vi "Butterfly_PullDown RCV_TTR.vi"(0 "Semiconductor Module Context":T2, 1 "RFPins":string[](array[string]), 3 "R Thresholds":dbl[](array[numeric]), 4 "Capacitance":bool=TRUE, 5 "error in (no error)":errorcluster, 6 "VNAs Measurement Parameters":T1, 7 "Start_v":dbl=10.0 format="%#_13g", 8 "C_TH_Delta":dbl=2.0, 9 "Stop_v":dbl=41.0 format="%#_13g", 10 "PD_Pin":string="SMU_PD", 11 "Step_v":dbl=1.0) -> (14 "Semiconductor Module Context Out":T2, 19 "error out":errorcluster)   [LabVIEW 2013]
uses:
  <vilib>/NI_TestStand_SemiconductorModule/NI_TestStand_Semiconductor_Module.lvlibp/PinMap/General/SemiconductorModuleContext.ctl
  VNA/VNAs Measurement Parameters.ctl
  <instrlib>/niDCPower/nidcpower.llb/niDCPower Wait For Event - Event.ctl
  <vilib>/NI_TestStand_SemiconductorModule/NI_TestStand_Semiconductor_Module.lvlibp/PinMap/DC Power/PinToNIDCPowerSession.vi
  <vilib>/NI_TestStand_SemiconductorModule/NI_TestStand_Semiconductor_Module.lvlibp/PinMap/DC Power/PinsToNIDCPowerSessions.vi
  <vilib>/NI_TestStand_SemiconductorModule/NI_TestStand_Semiconductor_Module.lvlibp/PinMap/General/Publish/PublishDataDoubleFunctionalTest.vi
  <vilib>/NI_TestStand_SemiconductorModule/NI_TestStand_Semiconductor_Module.lvlibp/PinMap/General/Publish/PublishDataDouble2D.vi
  <vilib>/NI_TestStand_SemiconductorModule/NI_TestStand_Semiconductor_Module.lvlibp
  VNA/Pin Map API/VNA Custom Instrument.lvlib
panel:
  in  "current level":dbl=0.01 format="%_6p"
  out "VPIs 2":dbl[](array[numeric])
  out "VRLs 2":dbl[](array[numeric])
  out "S0 steps":dbl[](array[numeric]) format="%#_3g"
  out "S1 steps":dbl[](array[numeric]) format="%#_3g"
  out "S2 steps":dbl[](array[numeric]) format="%#_3g"
  out "S3 steps":dbl[](array[numeric]) format="%#_3g"
  out "appended array":dbl[][](array[numeric]) format="%#_3g"
  out "VPIs":dbl[][](array[numeric]) format="%#_3g"
  out "VRLs":dbl[][](array[numeric]) format="%#_3g"
  out "C_Free":dbl[](array[numeric])
  out "Full R Array":dbl[][][](array[numeric])
  out "step":i32
  out "sites and pins loop iter":i32
  out "BF values":dbl[](array[numeric])
  out "BF Names":string[](array[string])
  out "R Array":dbl[](array[numeric])
  out "BFSamples":i32
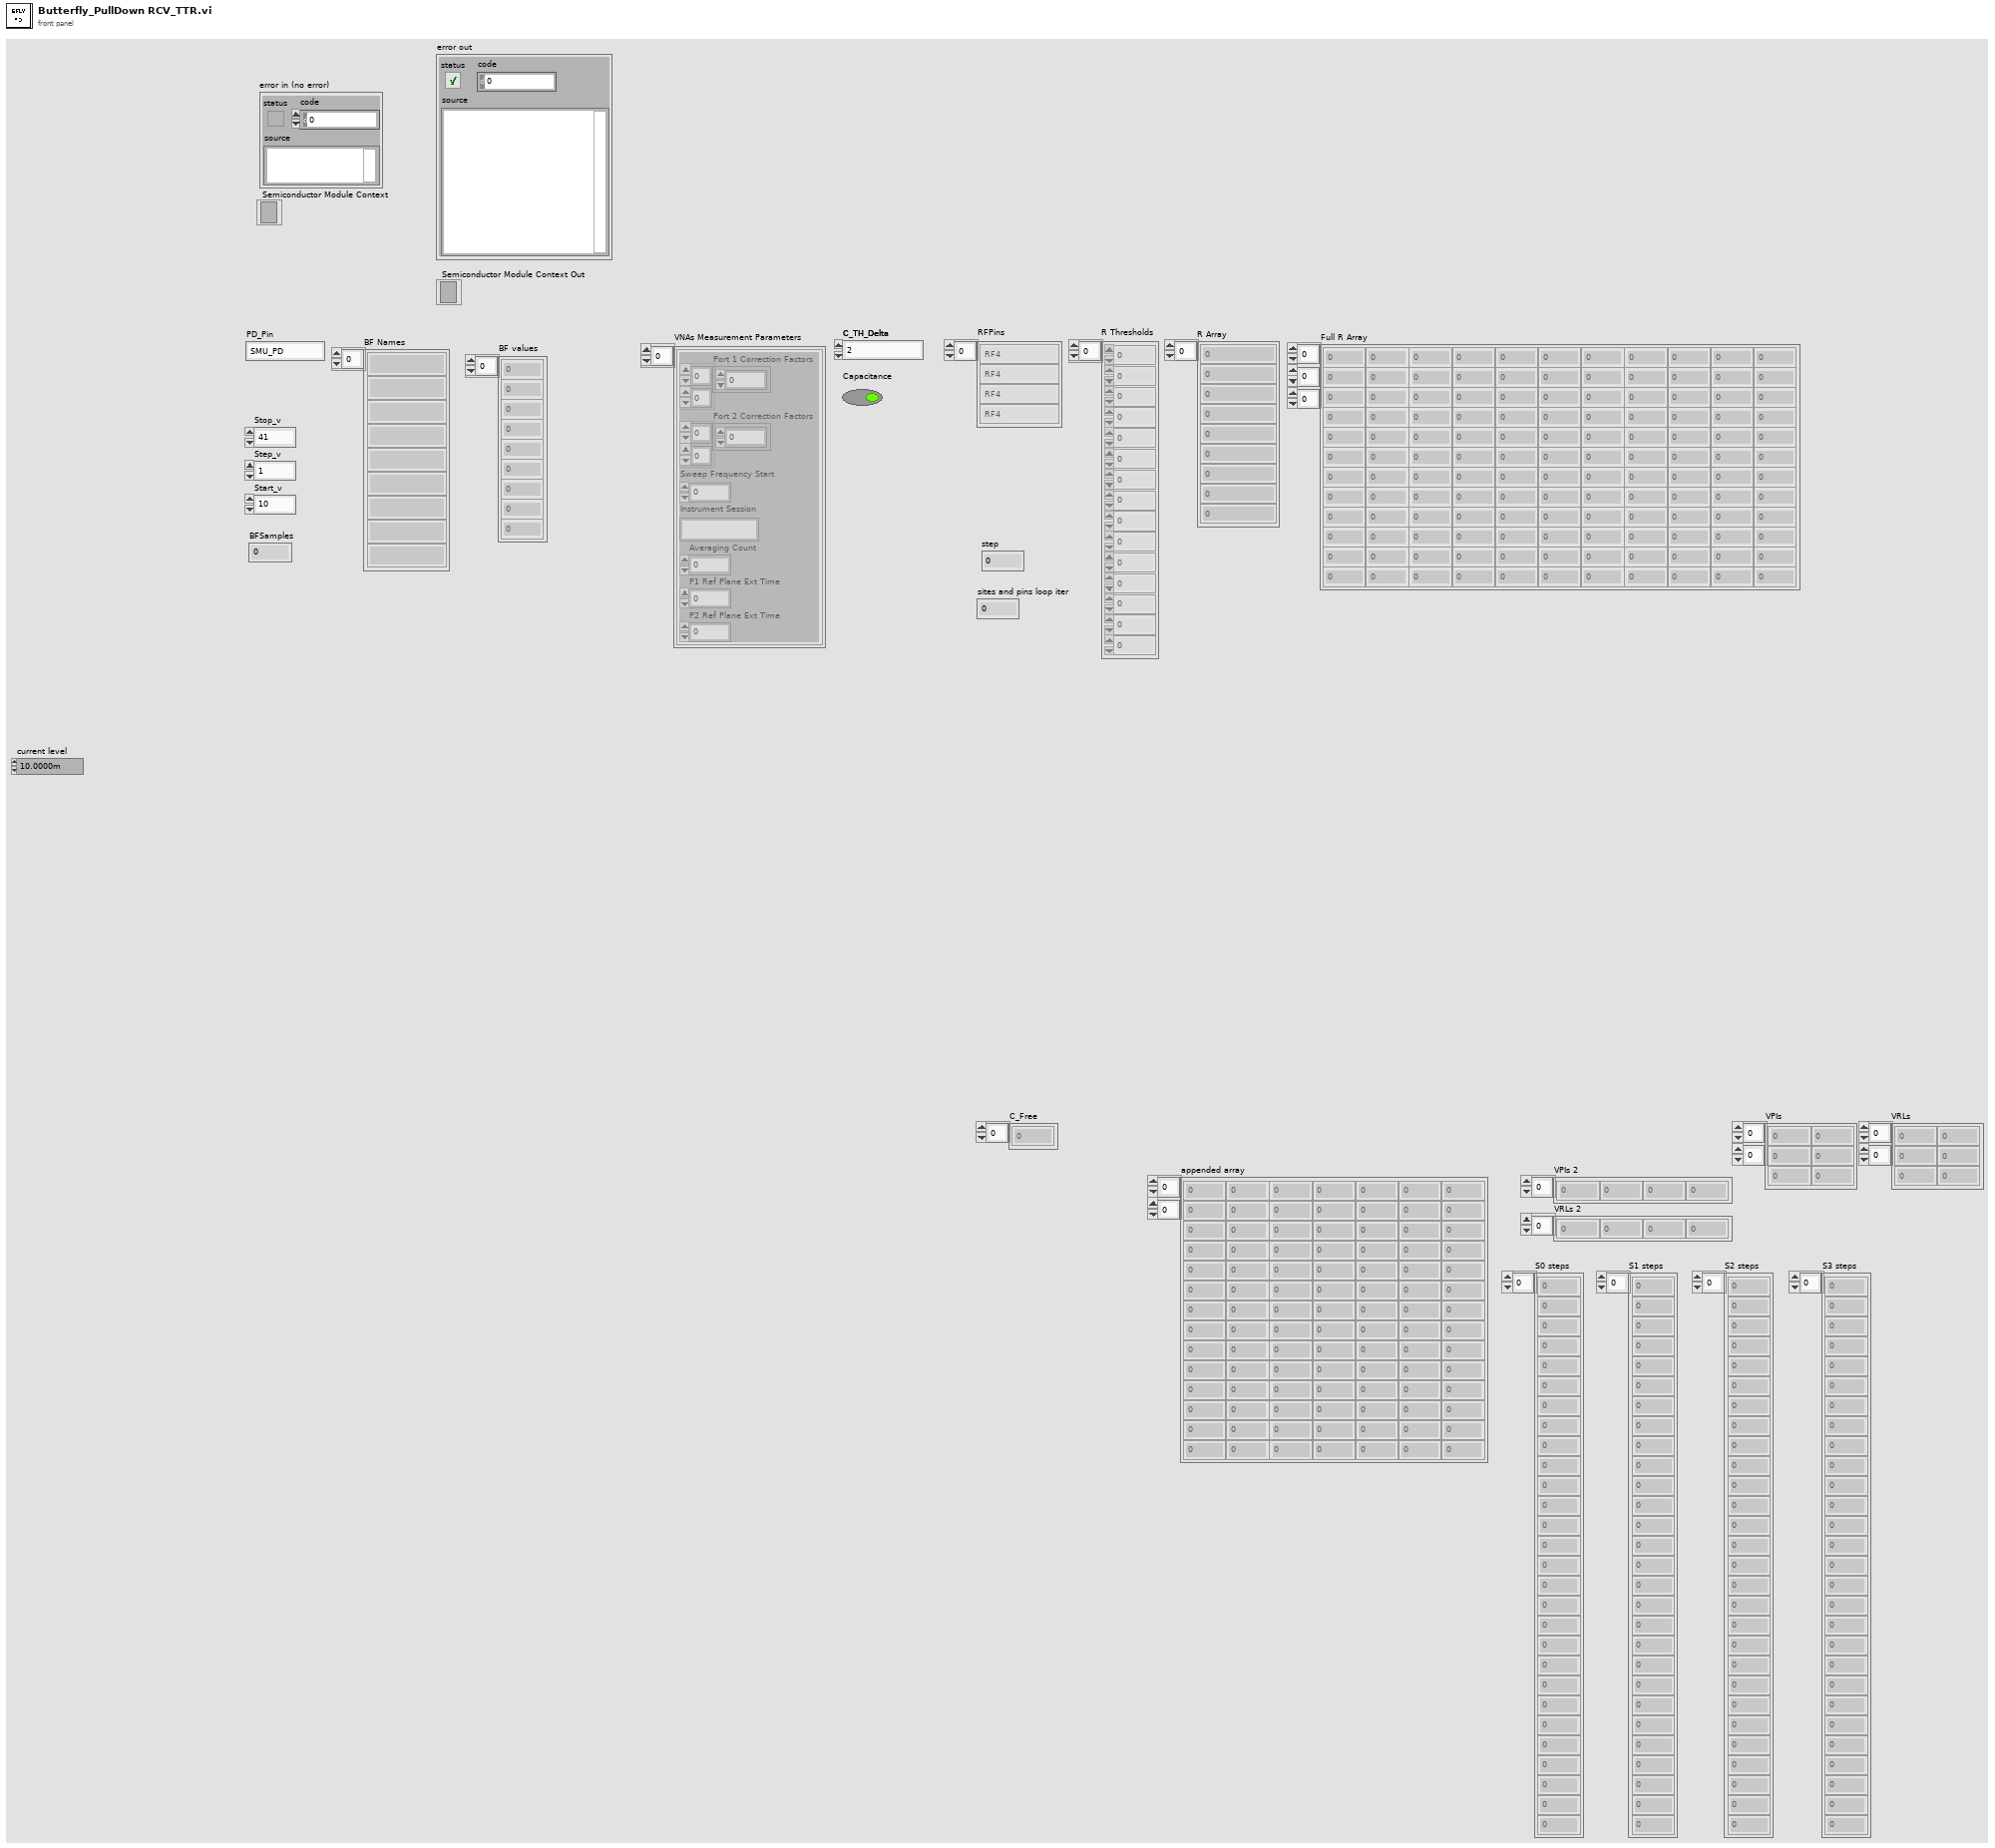
[diagram p1: front panel]
types:
  T1 = typedef "VNAs Measurement Parameters.ctl" = cluster{"Port 1 Correction Factors":cdb[][], "Port 2 Correction Factors":cdb[][], "Sweep Frequency Start":dbl, "Instrument Session":string, "Averaging Count":i32, "P1 Ref Plane Ext Time":dbl, "P2 Ref Plane Ext Time":dbl}[]
  T2 = typedef "NI_TestStand_Semiconductor_Module.lvlibp/SemiconductorModuleContext.ctl" = refnum<k7>
  T3 = typedef "niDCPower Wait For Event - Event.ctl" = i32
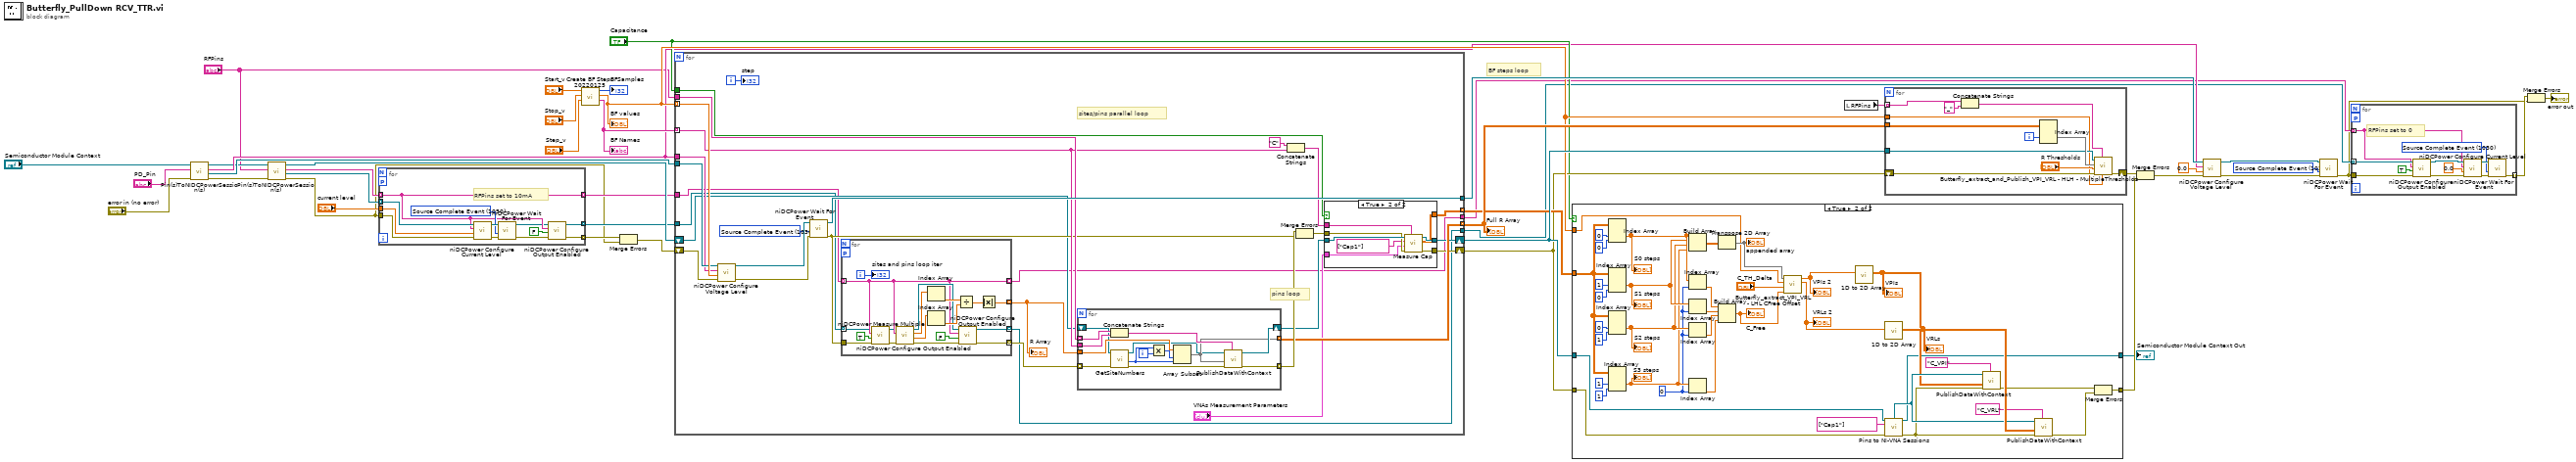
[diagram p0: block diagram]
diagram:
  w35 = T3 1030 items=["Source Complete Event"=1030, "Measure Complete Event"=1031, "Sequence Iteration Complete Event"=1032, "Sequence Engine Done Event"=1033, "Pulse Complete Event"=1051, "Ready For Pulse Trigger Event"=1052] ("event")
  # "BF steps loop"
  n1 = call-poly <vilib>:"Pin(s)ToNIDCPowerSession(s).vi"("error in (no error)"="error in (no error)", "Pin"="PD_Pin", "Semiconductor Module Context"="Semiconductor Module Context") -> ("error out"=w17:errorcluster, "Instrument Session"=w19:refnum<k15>, "Channel List"=w18:string, "Semiconductor Module Context Out"=w16:T2)  [unwired: 4 in, 1 out]
  n2 = call-poly <vilib>:"Pin(s)ToNIDCPowerSession(s).vi"("error in (no error)"=w17, "Pins"="RFPins", "Semiconductor Module Context"=w16) -> ("error out"=w1:errorcluster, "Instrument Sessions"=w13:refnum<k15>[], "Channel Lists"=w12:string[], "Semiconductor Module Context Out"=w15:T2)  [unwired: 4 in, 1 out]
  n3 = for {
    tunnel: w13 -> [w53] mode=indexing
    tunnel: w12 -> [w46] mode=indexing
    tunnel: "current level" -> [w50]
    tunnel: [w47] -> w9 mode=indexing
    tunnel: [w46] -> w10 mode=indexing
    workers-P: _ -> [_]
    tunnel: w1 -> [w52]
    tunnel: [w49] -> w2 mode=indexing
    w51 = T3 1030 items=["Source Complete Event"=1030, "Measure Complete Event"=1031, "Sequence Iteration Complete Event"=1032, "Sequence Engine Done Event"=1033, "Pulse Complete Event"=1051, "Ready For Pulse Trigger Event"=1052] ("event")
    # "RFPins set to 10mA"
    n4 = call <instrlib>:"niDCPower Configure Current Level.vi"("error in (no error)"=w52, "current level"=w50, "channel name"=w46, "instrument handle"=w53) -> ("error out"=w55:errorcluster, "instrument handle out"=w54:refnum<k15>)  [unwired: 6 in]
    n5 = call <instrlib>:"niDCPower Wait For Event.vi"("error in (no error)"=w55, "event"=w51, "instrument handle"=w54) -> ("error out"=w44:errorcluster, "instrument handle out"=w45:refnum<k15>)  [unwired: 7 in]
    n6 = call <instrlib>:"niDCPower Configure Output Enabled.vi"("error in (no error)"=w44, "output enabled"=FALSE, "channel name"=w46, "instrument handle"=w45) -> ("error out"=w49:errorcluster, "instrument handle out"=w47:refnum<k15>)  [unwired: 6 in]
  }
  n7 = call "Create BF Steps 20220125.vi"("Step_v"="Step_v", "Stop_v"="Stop_v", "Start_v"="Start_v") -> ("BF Names"=w34:string[], "BF values"=w29:dbl[], "BFSamples"=→"BFSamples":i32)  [unwired: 6 in]
  "BF Names" <- w34
  "BF values" <- w29
  n8 = Merge Errors(w2, w1) -> (w3:errorcluster)
  n9 = for {
    shift-right: [w69] -> w28
    shift-left: w3 -> [w82]
    tunnel: w29 -> [w81] mode=indexing
    tunnel: w19 -> [w80]
    tunnel: [w79] -> w38
    shift-right: [w64] -> w31
    shift-left: w15 -> [w60]
    tunnel: "RFPins" -> [w76]
    tunnel: w34 -> [w67] mode=indexing
    tunnel: [w74] -> w32 mode=indexing
    tunnel: "Capacitance" -> [w65]
    tunnel: [w63] -> w30 mode=indexing
    tunnel: w18 -> [w62]
    tunnel: w10 -> [w59]
    tunnel: w9 -> [w58]
    tunnel: [w57] -> w8
    tunnel: [w56] -> w7
    i -> [w78]
    w84 = T3 1030 items=["Source Complete Event"=1030, "Measure Complete Event"=1031, "Sequence Iteration Complete Event"=1032, "Sequence Engine Done Event"=1033, "Pulse Complete Event"=1051, "Ready For Pulse Trigger Event"=1052] ("event")
    # "pins loop"
    # "sites/pins parallel loop"
    n10 = call <instrlib>:"niDCPower Configure Voltage Level.vi"("error in (no error)"=w82, "voltage level"=w81, "channel name"=w62, "instrument handle"=w80) -> ("error out"=w83:errorcluster, "instrument handle out"=w85:refnum<k15>)  [unwired: 6 in]
    n11 = call <instrlib>:"niDCPower Wait For Event.vi"("error in (no error)"=w83, "event"=w84, "instrument handle"=w85) -> ("error out"=w61:errorcluster, "instrument handle out"=w79:refnum<k15>)  [unwired: 7 in]
    n12 = for {
      tunnel: w61 -> [w120]
      tunnel: [w122] -> w75 mode=indexing
      tunnel: [w117] -> w73 mode=indexing
      workers-P: _ -> [_]
      tunnel: w59 -> [w114] mode=indexing
      tunnel: w58 -> [w113] mode=indexing
      tunnel: [w115] -> w57 mode=indexing
      tunnel: [w114] -> w56 mode=indexing
      i -> [w121]
      n13 = call <instrlib>:"niDCPower Configure Output Enabled.vi"("error in (no error)"=w120, "output enabled"=TRUE, "channel name"=w114, "instrument handle"=w113) -> ("error out"=w119:errorcluster, "instrument handle out"=w110:refnum<k15>)  [unwired: 6 in]
      n14 = call <instrlib>:"niDCPower Measure Multiple.vi"("error in (no error)"=w119, "channel name"=w114, "instrument handle"=w110) -> ("error out"=w118:errorcluster, "current measurements"=w123:dbl[], "voltage measurements"=w124:dbl[], "instrument handle out"=w116:refnum<k15>)  [unwired: 5 in]
      n15 = Index Array(array=w124) -> (element=w126:dbl)  [unwired: 1 in]
      n16 = Index Array(array=w123) -> (element=w125:dbl)  [unwired: 1 in]
      n17 = Divide(x=w126, y=w125) -> (x/y=w127:dbl)
      n18 = call <instrlib>:"niDCPower Configure Output Enabled.vi"("error in (no error)"=w118, "output enabled"=FALSE, "channel name"=w114, "instrument handle"=w116) -> ("error out"=w117:errorcluster, "instrument handle out"=w115:refnum<k15>)  [unwired: 6 in]
      n19 = Absolute Value(x=w127) -> (abs(x)=w122:dbl)
      "sites and pins loop iter" <- w121
    }
    "R Array" <- w75
    n20 = for {
      tunnel: [w104] -> w77 mode=indexing
      tunnel: w76 -> [w108] mode=indexing
      tunnel: w75 -> [w105]
      tunnel: w67 -> [w107]
      shift-right: [w102] -> w72
      shift-left: w60 -> [w99]
      tunnel: [w101] -> w74 mode=indexing
      tunnel: w73 -> [w96] mode=indexing
      i -> [w109]
      n21 = Concatenate Strings(w108, w107) -> (w103:string)
      n22 = call <vilib>:"GetSiteNumbers.vi"("error in (no error)"=w96, "Semiconductor Module Context"=w99) -> ("error out"=w100:errorcluster, "Number Of Sites"=w97:i32, "Semiconductor Module Context Out"=w98:T2)  [unwired: 6 in, 1 out]
      n23 = Multiply(x=w97, y=w109) -> (x*y=w106:i32)
      n24 = Array Subset(array=w105, index=w106, length=w97) -> (w101:dbl[])
      n25 = call-poly <vilib>:"PublishDataWithContext.vi"("Published Data Id"=w103, "error in (no error)"=w100, "Data In"=w101, "Semiconductor Module Context"=w98) -> ("error out"=w104:errorcluster, "Semiconductor Module Context Out"=w102:T2)  [unwired: 6 in]
    }
    n26 = Concatenate Strings("C" ("string"), w67) -> (w66:string)
    n27 = Merge Errors(w77, w61) -> (w70:errorcluster)
    n28 = case shown="True" w65 {
      tunnel: w72 -> [w87 w95]
      tunnel: [w87 w94] -> w64
      tunnel: [w86 w92] -> w69
      tunnel: w66 -> [_ w88]
      tunnel: "VNAs Measurement Parameters" -> [_ w90]
      tunnel: [_ w91] -> w63
      tunnel: w70 -> [w86 w93]
      frame False {
      }
      frame True {
        n29 = call "Measure Cap.vi"("Measurement Id"=w88, "error in (no error)"=w93, "VNAs Measurement Parameters"=w90, "Pins"=string[] ["Cap1"] ("Capacitance Pins"), "Semiconductor Module Context"=w95) -> ("error out"=w92:errorcluster, "Multisite Cap Data"=w91:dbl[][], "Semiconductor Module Context Out"=w94:T2)  [unwired: 4 in]
      }
    }
    "step" <- w78
  }
  "Full R Array" <- w32
  n30 = case shown="True" "Capacitance" {
    tunnel: [w128 w148] -> w23
    tunnel: [w129 w166] -> w25
    tunnel: w31 -> [w128 w165]
    tunnel: w28 -> [w129 w161]
    tunnel: w29 -> [_ w133]
    tunnel: w30 -> [_ w152]
    frame False {
    }
    frame True {
      w141 = 0 ("index")
      n31 = Index Array(array=w152, index (dim 1)=0 ("disabled index (row)"), index (dim 2)=0 ("disabled index (col)")) -> (element=w145:dbl[])  [unwired: 1 in]
      "S0 steps" <- w145
      n32 = Index Array(array=w152, index (dim 1)=1 ("index (row)"), index (dim 2)=0 ("index (col)")) -> (element=w144:dbl[])  [unwired: 1 in]
      "S1 steps" <- w144
      n33 = Index Array(array=w152, index (dim 1)=0 ("index (row)"), index (dim 2)=1 ("index (col)")) -> (element=w143:dbl[])  [unwired: 1 in]
      "S2 steps" <- w143
      n34 = Index Array(array=w152, index (dim 1)=1 ("index (row)"), index (dim 2)=1 ("index (col)")) -> (element=w142:dbl[])  [unwired: 1 in]
      "S3 steps" <- w142
      n35 = Build Array(w145, w144, w143, w142) -> (w136:dbl[][])
      n36 = Index Array(array=w145, index=w141) -> (element=w140:dbl)
      n37 = Index Array(array=w144, index=w141) -> (element=w139:dbl)
      n38 = Index Array(array=w143, index=w141) -> (element=w138:dbl)
      n39 = Index Array(array=w142, index=w141) -> (element=w137:dbl)
      n40 = Transpose 2D Array(2D array=w136) -> (transposed array=w134:dbl[][])
      "appended array" <- w134
      n41 = Build Array(w140, w139, w138, w137) -> (w135:dbl[])
      "C_Free" <- w135
      n42 = call "Butterfly_extract_VPI_VRL - LHL CFree Offset.vi"("C_Free"=w135, "Delta"="C_TH_Delta", "Voltage Array"=w133, "Result Array In"=w134) -> ("VRLs"=w130:dbl[], "VPIs"=w131:dbl[])  [unwired: 6 in]
      "VPIs 2" <- w131
      "VRLs 2" <- w130
      n43 = call "1D to 2D Array.vi"("1D Array"=w131) -> ("2D Array"=w150:dbl[][])  [unwired: 10 in]
      "VPIs" <- w150
      n44 = call "1D to 2D Array.vi"("1D Array"=w130) -> ("2D Array"=w164:dbl[][])  [unwired: 10 in]
      "VRLs" <- w164
      n45 = call "Pins to NI-VNA Sessions.vi"("Semiconductor Module Context"=w165, "Pins"=string[] ["Cap1"] ("Capacitance Pins"), "error in (no error)"=w161) -> ("Pin Query Context"=w151:refnum<class "MultiplePinMultipleSessionQueryContext.lvclass">, "Semiconductor Module Context Out"=w148:T2, "error out"=w146:errorcluster)  [unwired: 8 in, 2 out]
      n46 = call-poly <vilib>:"PublishDataWithContext.vi"("Published Data Id"="C_VPI", "error in (no error)"=w146, "Data In"=w150, "Pin Query Context"=w151) -> ("error out"=w147:errorcluster)  [unwired: 6 in, 1 out]
      n47 = call-poly <vilib>:"PublishDataWithContext.vi"("Published Data Id"="C_VRL", "error in (no error)"=w146, "Data In"=w164, "Pin Query Context"=w151) -> ("error out"=w167:errorcluster)  [unwired: 6 in, 1 out]
      n48 = Merge Errors(w147, w167) -> (w166:errorcluster)
    }
  }
  "Semiconductor Module Context Out" <- w23
  n49 = local read "RFPins"() -> (w33:string[])
  n50 = for {
    tunnel: w33 -> [w172] mode=indexing
    tunnel: w32 -> [w177]
    shift-right: [w173] -> w26
    shift-left: w28 -> [w174]
    tunnel: w31 -> [w169]
    tunnel: w29 -> [w168]
    i -> [w178]
    n51 = Concatenate Strings(w172, "_" ("string")) -> (w170:string)
    n52 = Index Array(array=w177, index (dim 1)=w178) -> (element=w175:dbl[][])  [unwired: 2 in]
    n53 = call "Butterfly_extract_and_Publish_VPI_VRL - HLH - MultipleThresholds.vi"("Voltages Array"=w168, "ID Prefix"=w170, "error in (no error)"=w174, "Thresholds"="R Thresholds", "Result Array In"=w175, "Semiconductor Module Context"=w169) -> ("error out"=w173:errorcluster)  [unwired: 5 in]
  }
  n54 = Merge Errors(w26, w25) -> (w24:errorcluster)
  n55 = call <instrlib>:"niDCPower Configure Voltage Level.vi"("error in (no error)"=w24, "voltage level"=0.0, "channel name"=w18, "instrument handle"=w38) -> ("error out"=w37:errorcluster, "instrument handle out"=w36:refnum<k15>)  [unwired: 6 in]
  n56 = call <instrlib>:"niDCPower Wait For Event.vi"("error in (no error)"=w37, "event"=w35, "instrument handle"=w36) -> ("error out"=w4:errorcluster)  [unwired: 7 in, 1 out]
  n57 = for {
    tunnel: w8 -> [w182] mode=indexing
    tunnel: w7 -> [w180] mode=indexing
    workers-P: _ -> [_]
    tunnel: w4 -> [w184]
    tunnel: [w186] -> w6 mode=indexing
    w185 = T3 1030 items=["Source Complete Event"=1030, "Measure Complete Event"=1031, "Sequence Iteration Complete Event"=1032, "Sequence Engine Done Event"=1033, "Pulse Complete Event"=1051, "Ready For Pulse Trigger Event"=1052] ("event")
    # "RFPins set to 0"
    n58 = call <instrlib>:"niDCPower Configure Output Enabled.vi"("error in (no error)"=w184, "output enabled"=TRUE, "channel name"=w180, "instrument handle"=w182) -> ("error out"=w183:errorcluster, "instrument handle out"=w181:refnum<k15>)  [unwired: 6 in]
    n59 = call <instrlib>:"niDCPower Configure Current Level.vi"("error in (no error)"=w183, "current level"=0.0, "channel name"=w180, "instrument handle"=w181) -> ("error out"=w189:errorcluster, "instrument handle out"=w188:refnum<k15>)  [unwired: 6 in]
    n60 = call <instrlib>:"niDCPower Wait For Event.vi"("error in (no error)"=w189, "event"=w185, "instrument handle"=w188) -> ("error out"=w186:errorcluster)  [unwired: 7 in, 1 out]
  }
  n61 = Merge Errors(w6, w4) -> (→"error out":errorcluster)
